vi "FPGA Main.vi"() -> ()   [LabVIEW 2010]
uses:
  Motor Control/Motor Encoder Global.vi
  Motor Control/Motor Output Global.vi
  Motor Control/Inner Control/Drive Control Global DO NOT MODIFY!.vi
  behaviors/driveable path/drivable paths global.vi
  Deleteme/line driveable paths global.vi
panel:
  out "current state":enum16{"Human Control", "Autonomous"}(ring)
  in  "desired state":enum16{"Human Control", "Autonomous"}(ring)
  out "line driveable path lengths":u16[](array[numeric])
  in  "line proximity":i16=100
  in  "Auton Steering Position":i32
  in  "Auton Steering Enable":bool
  in  "Auton Drive Enable":bool
  in  "obstacle proximity":i16=400
  out "Steering Position":i32
  out "Drive Speed Current":fxp<+/-,18,8> format="%.13g"
  out "Drive Enabled?":bool
  out "Steering Enabled?":bool
  out "obstacle driveable path lengths":u16[](array[numeric])
  in  "Autonomous Drive Current":fxp<+/-,18,8>
  in  "Steering Position Offset":i32
  out "Drive Encoder ft/sec":fxp<+/-,18,8>
  in  "Enable Drive":bool
  in  "Drive Speed Current (1-3.5)":fxp<+/-,18,8>
  in  "Steering Proportional Control Feedback Gain":fxp<+/-,20,5>
  in  "Enable Steering":bool
  in  "Steering Position Target":i32
  # "Athena FPGA Main"
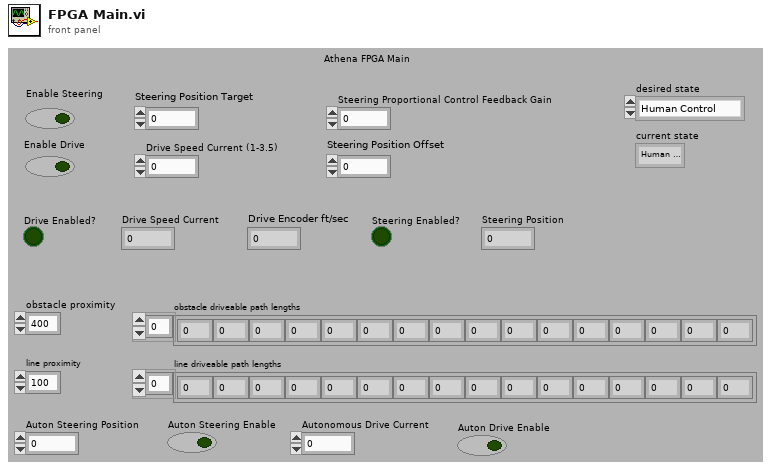
[diagram p1: front panel]
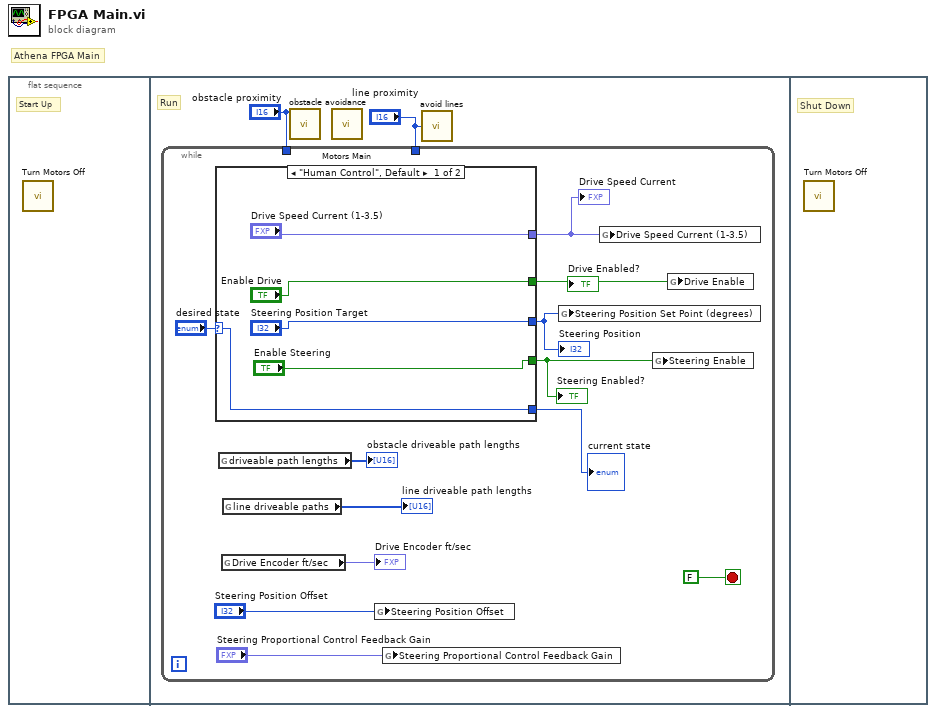
[diagram p0: block diagram]
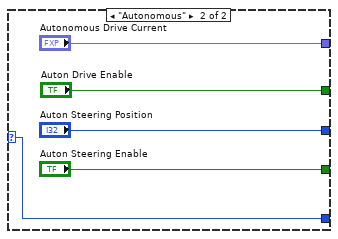
[diagram p2: hidden frame]
diagram:
  # "Athena FPGA Main"
  n1 = flat-sequence {
    frame #0 {
      # "Start Up"
      n2 = call "Turn Motors Off.vi"() -> ()  [unwired: 1 in]
    }
    frame #1 {
      # "Run"
      n3 = while {
        tunnel: "obstacle proximity" -> [_]
        tunnel: "line proximity" -> [_]
        stop <- FALSE stop-if-true
        n4 = case shown="\"Human Control\", Default" "desired state" {
          selector: "desired state" -> [w15 w20]
          tunnel: ["Steering Position Target" "Auton Steering Position"] -> w7
          tunnel: ["Enable Drive" "Auton Drive Enable"] -> w12
          tunnel: ["Enable Steering" "Auton Steering Enable"] -> w11
          tunnel: ["Drive Speed Current (1-3.5)" "Autonomous Drive Current"] -> w10
          tunnel: [w15 w20] -> w3
          frame "Human Control", Default {
          }
          frame "Autonomous" {
          }
        }
        "Steering Enabled?" <- w11
        "Drive Enabled?" <- w12
        "Drive Speed Current" <- w10
        "Steering Position" <- w7
        "current state" <- w3
        n5 = global read "drivable paths global.vi" "driveable path lengths"() -> (→"obstacle driveable path lengths":u16[])
        n6 = global read "Drive Control Global DO NOT MODIFY!.vi" "Drive Encoder ft/sec"() -> (→"Drive Encoder ft/sec":fxp<+/-,18,8>)
        n7 = global read "line driveable paths global.vi" "line driveable paths"() -> (→"line driveable path lengths":u16[])
        n8 = global write "Motor Encoder Global.vi" "Steering Position Offset"("Steering Position Offset") -> ()
        n9 = global write "Motor Encoder Global.vi" "Steering Proportional Control Feedback Gain"("Steering Proportional Control Feedback Gain") -> ()
        n10 = global write "Motor Encoder Global.vi" "Steering Position Set Point (degrees)"(w7) -> ()
        n11 = global write "Motor Encoder Global.vi" "Drive Speed Current (1-3.5)"(w10) -> ()
        n12 = global write "Motor Output Global.vi" "Steering Enable"(w11) -> ()
        n13 = global write "Motor Output Global.vi" "Drive Enable"(w12) -> ()
      }
      n14 = call "obstacle avoidance.vi"("allowed proximity squared"="obstacle proximity") -> ()  [unwired: 11 in]
      n15 = call "Motors Main.vi"() -> ()  [unwired: 1 in]
      n16 = call "avoid lines.vi"("allowed proximity squared"="line proximity") -> ()
    }
    frame #2 {
      # "Shut Down"
      n17 = call "Turn Motors Off.vi"() -> ()  [unwired: 1 in]
    }
  }
